vi "Do.vi"(8 "error in (no error)":errorcluster, 10 "Actor in":refnum<class "Actor.lvclass">, 11 "Send Results Object":refnum<class "Send Results Object.lvclass">) -> (0 "error out":errorcluster, 2 "Actor out":refnum<class "Actor.lvclass">)   [LabVIEW 2016, in "Controller Actor.lvlib" / "Send Results Object.lvclass"]
uses:
  <userlib>/Common Components/Controller/Messages/Send Results Object/Send Results Object.lvclass
  <vilib>/ActorFramework/Actor/Actor.lvclass
  <userlib>/Common Components/Controller/Controller.lvclass
  C:/Program Files (x86)/National Instruments/LabVIEW 2016/vi.lib/ActorFramework/Actor/Actor.lvclass
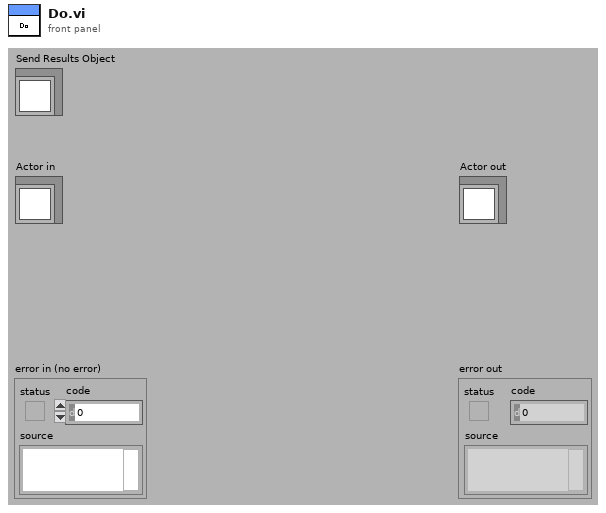
[diagram p1: front panel]
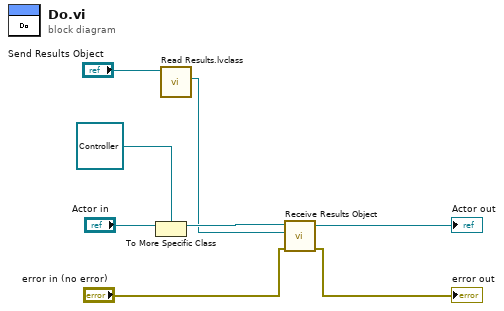
[diagram p0: block diagram]
diagram:
  n1 = To More Specific Class(target class=refnum<class "Controller.lvclass"> refnum ("Controller.lvclass"), reference="Actor in") -> (specific class reference=w5:refnum<class "Controller.lvclass">)  [unwired: 1 in, 1 out]
  n2 = call <userlib>:"Read Results.lvclass.vi"("Send Results Object in"="Send Results Object") -> ("Results.lvclass"=w3:refnum<class "Results.lvclass">)  [unwired: 8 in, 2 out]
  n3 = call-dynamic "Receive Results Object.vi"("error in (no error)"="error in (no error)", "Results.lvclass"=w3, "Controller in"=w5) -> ("error out"=→"error out":errorcluster, "Controller out"=→"Actor out":refnum<class "Controller.lvclass">)  [unwired: 7 in]
